vi "CAN Send Msg.vi"(7 "SendMsgNum":u32, 9 "pCanSendMsg":T1, 10 "CANIndex":u8, 11 "DevIndex":i32) -> (3 "function return":i32)   [LabVIEW 2010, in "usb2can.lvlib"]
doc: "int WINAPI CAN_SendMsg(int DevIndex, unsigned char CANIndex, PCAN_MSG pCanSendMsg,unsigned int SendMsgNum);"
uses:
  usb2can.lvlib
  USB2XXX.dll
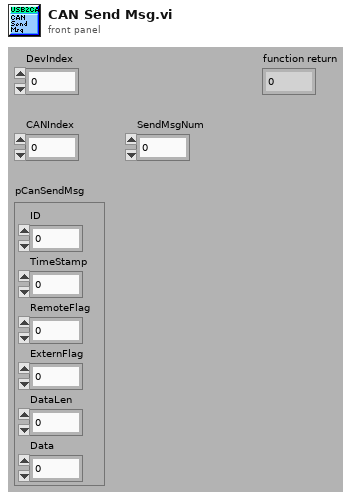
[diagram p1: front panel]
types:
  T1 = cluster{"ID":u32, "TimeStamp":u32, "RemoteFlag":u8, "ExternFlag":u8, "DataLen":u8, "Data":u8}
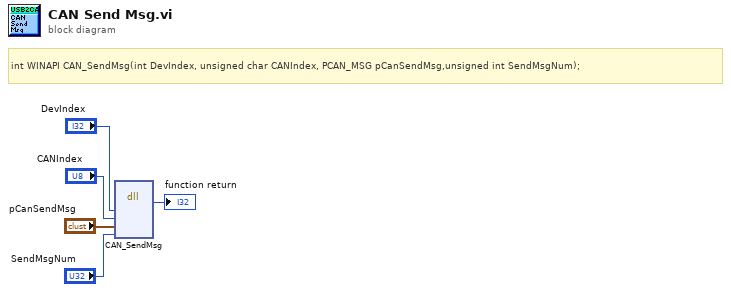
[diagram p0: block diagram]
diagram:
  # "int WINAPI CAN_SendMsg(int DevIndex, unsigned char CANIndex, PCAN_MSG pCanSendMsg,unsigned int SendMsgNum);"
  n1 = dll-call lib="F:/OtherWork/STM32/USB2XXX_Example/trunk/Labview/PublicFiles/usb2can/USB2XXX.*" fn="CAN_SendMsg"("DevIndex"="DevIndex", "CANIndex"="CANIndex", "pCanSendMsg"="pCanSendMsg", "SendMsgNum"="SendMsgNum") -> (→"function return":i32)  [unwired: 7 in, 2 out]
